vi "ContextManager.FGV.vi"(10 "error in":errorcluster, 11 "action":T1) -> (2 "error out":errorcluster, 3 "context":refnum<class "zmq_context.lvclass">)   [LabVIEW 2019, in "RemoteControl.ZMQ.lvlib" / "ZMQ.ContextManager.lvlib"]
uses:
  ZMQ.ContextManager.lvlib
  <vilib>/addons/zeromq/zmq_context.lvclass
  Typedefs/Action--enum.ctl
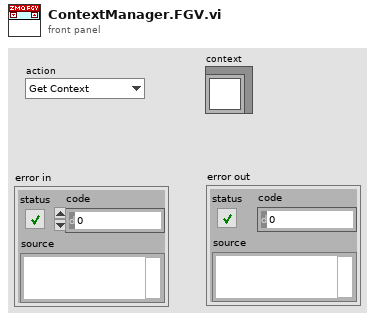
[diagram p1: front panel]
types:
  T1 = typedef "RemoteControl.ZMQ.lvlib/ZMQ.ContextManager.lvlib/Action--enum.ctl" = enum16{"Get Context", "Release Context", "Socket Opened", "Socket Closed", "Force Cleanup"}
  T2 = typedef "RemoteControl.ZMQ.lvlib/ZMQ.ContextManager.lvlib/Context--DVR.ctl" = refnum<data-value>
  T3 = typedef "RemoteControl.ZMQ.lvlib/ZMQ.ContextManager.lvlib/Context--Cluster.ctl" = cluster{"context":refnum<class "zmq_context.lvclass">, "context counter":u32, "socket counter":u32}
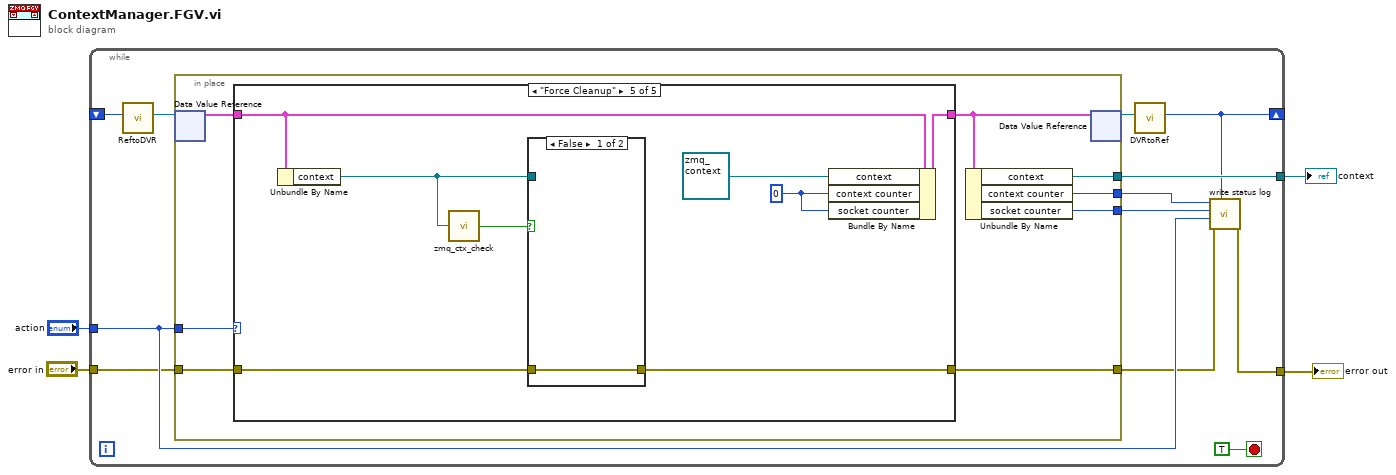
[diagram p0: block diagram]
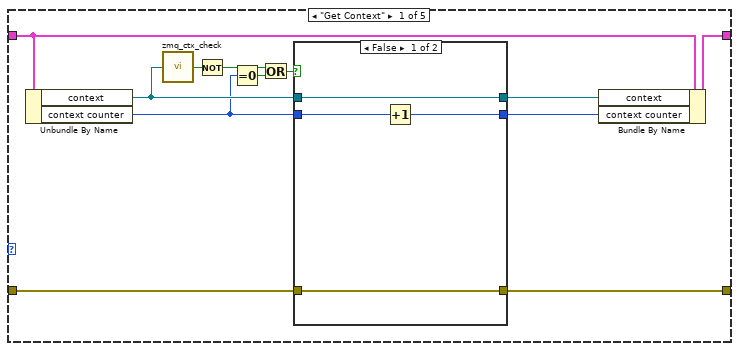
[diagram p2: hidden frame]
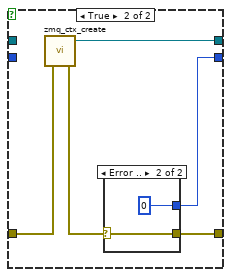
[diagram p3: hidden frame]
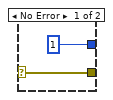
[diagram p4: hidden frame]
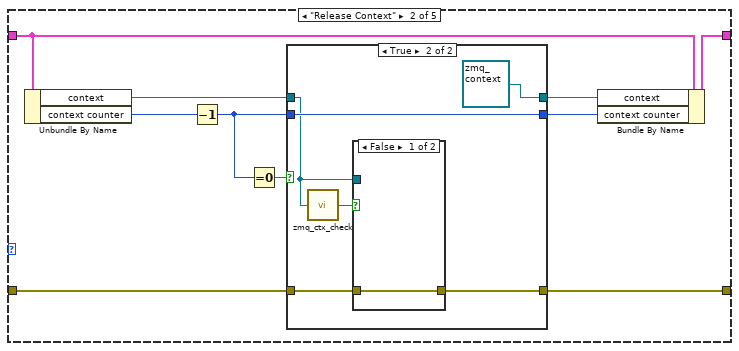
[diagram p5: hidden frame]
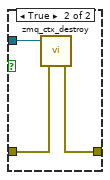
[diagram p7: hidden frame]
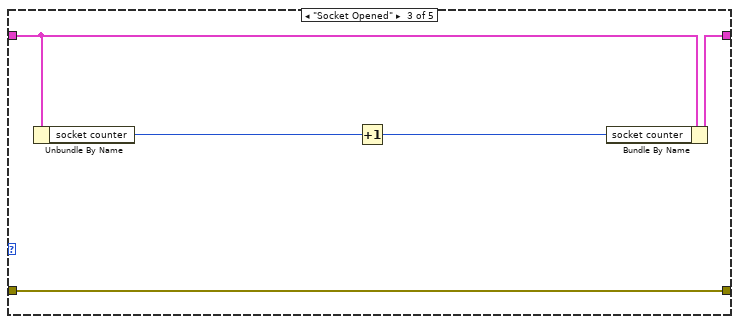
[diagram p8: hidden frame]
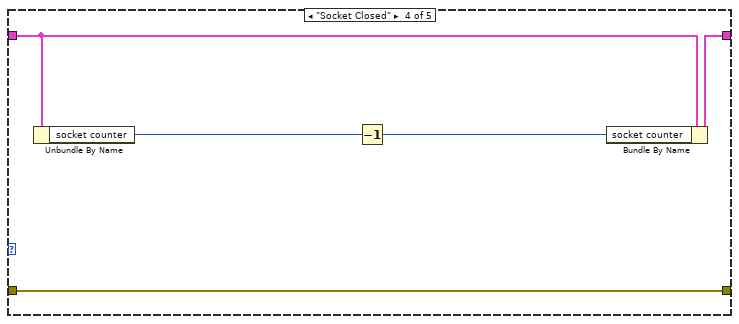
[diagram p9: hidden frame]
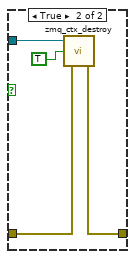
[diagram p10: hidden frame]
diagram:
  n1 = while {
    tunnel: "action" -> [w8]
    shift-right: [w11] -> _
    shift-left: _ -> [w15]
    tunnel: [w12] -> w3
    tunnel: "error in" -> [w7]
    tunnel: [w5] -> w1
    stop <- TRUE stop-if-true
    n2 = call "ReftoDVR.vi"("Ref"=w15) -> ("DVR"=w13:T2)  [unwired: 10 in]
    n3 = in-place {
      in-place-border: [w24] -> w6
      in-place-border: w8 -> [w23]
      in-place-border: [w20] -> w12
      in-place-border: [w19] -> w10
      in-place-border: [w18] -> w9
      in-place-border: w7 -> [w17]
      n4 = in-place-dvr #1(w13) -> (w22:T3)  [unwired: 1 out]
      n5 = case shown="\"Force Cleanup\"" w23 {
        tunnel: w17 -> [w36 w59 w77 w82 w83]
        tunnel: [w35 w58 w77 w82 w90] -> w24
        tunnel: w22 -> [w29 w53 w76 w81 w87]
        tunnel: [w25 w52 w73 w78 w86] -> w21
        frame "Get Context" {
          n6 = Unbundle By Name(w29) -> ("context"=w30:refnum<class "zmq_context.lvclass">, "context counter"=w26:u32)
          n7 = call <vilib>:"zmq_ctx_check.vi"("context in"=w30) -> ("valid?"=w34:bool)
          n8 = Not(x=w34) -> (.not. x?=w31:bool)
          n9 = Equal To 0?(x=w26) -> (x = 0?=w32:bool)
          n10 = Or(x=w31, y=w32) -> (x .or. y?=w33:bool)
          n11 = case shown="False" w33 {
            tunnel: [w37 w45] -> w28
            tunnel: w36 -> [w40 w44]
            tunnel: [w40 w41] -> w35
            tunnel: w26 -> [w39 _]
            tunnel: [w38 w43] -> w27
            tunnel: w30 -> [w37 _]
            frame False {
              n12 = Increment(x=w39) -> (x+1=w38:u32)
            }
            frame True {
              n13 = call <vilib>:"zmq_ctx_create.vi"("error in"=w44) -> ("error out"=w42:errorcluster, "context out"=w45:refnum<class "zmq_context.lvclass">)  [unwired: 3 in]
              n14 = case shown="Error .." w42 {
                selector: w42 -> [w46 w48]
                tunnel: [u32 1 u32 0] -> w43
                tunnel: [w46 w48] -> w41
                frame No Error {
                }
                frame Error {
                }
              }
            }
          }
          n15 = Bundle By Name(cluster=w29, "context"=w28, "context counter"=w27) -> (w25:T3)
        }
        frame "Release Context" {
          n16 = Unbundle By Name(w53) -> ("context"=w50:refnum<class "zmq_context.lvclass">, "context counter"=w51:u32)
          n17 = Decrement(x=w51) -> (x-1=w55:u32)
          n18 = Equal To 0?(x=w55) -> (x = 0?=w57:bool)
          n19 = case shown="True" w57 {
            tunnel: w59 -> [w62 w68]
            tunnel: [w62 w67] -> w58
            tunnel: [w61 refnum<class "zmq_context.lvclass"> refnum ("context out")] -> w54
            tunnel: w50 -> [w61 w63]
            tunnel: [w60 w64] -> w56
            tunnel: w55 -> [w60 w64]
            frame False {
            }
            frame True {
              n20 = call <vilib>:"zmq_ctx_check.vi"("context in"=w63) -> ("valid?"=w66:bool)
              n21 = case shown="False" w66 {
                tunnel: w68 -> [w69 w72]
                tunnel: [w69 w71] -> w67
                tunnel: w63 -> [_ w70]
                frame False {
                }
                frame True {
                  n22 = call <vilib>:"zmq_ctx_destroy.vi"("error in"=w72, "context in"=w70) -> ("error out"=w71:errorcluster)  [unwired: 3 in]
                }
              }
            }
          }
          n23 = Bundle By Name(cluster=w53, "context"=w54, "context counter"=w56) -> (w52:T3)
        }
        frame "Socket Opened" {
          n24 = Unbundle By Name(w76) -> ("socket counter"=w75:u32)
          n25 = Increment(x=w75) -> (x+1=w74:u32)
          n26 = Bundle By Name(cluster=w76, "socket counter"=w74) -> (w73:T3)
        }
        frame "Socket Closed" {
          n27 = Unbundle By Name(w81) -> ("socket counter"=w80:u32)
          n28 = Decrement(x=w80) -> (x-1=w79:u32)
          n29 = Bundle By Name(cluster=w81, "socket counter"=w79) -> (w78:T3)
        }
        frame "Force Cleanup" {
          w85 = u32 0
          n30 = Unbundle By Name(w87) -> ("context"=w84:refnum<class "zmq_context.lvclass">)
          n31 = call <vilib>:"zmq_ctx_check.vi"("context in"=w84) -> ("valid?"=w89:bool)
          n32 = case shown="False" w89 {
            tunnel: w83 -> [w91 w95]
            tunnel: [w91 w94] -> w90
            tunnel: w84 -> [_ w92]
            frame False {
            }
            frame True {
              n33 = call <vilib>:"zmq_ctx_destroy.vi"("error in"=w95, "reap? (F)"=TRUE, "context in"=w92) -> ("error out"=w94:errorcluster)  [unwired: 2 in]
            }
          }
          n34 = Bundle By Name(cluster=w87, "context"=refnum<class "zmq_context.lvclass"> refnum ("context out"), "context counter"=w85, "socket counter"=w85) -> (w86:T3)
        }
      }
      n35 = Unbundle By Name(w21) -> ("context"=w20:refnum<class "zmq_context.lvclass">, "context counter"=w19:u32, "socket counter"=w18:u32)
      n36 = in-place-dvr #1(w21) -> (w14:T2)  [unwired: 1 out]
    }
    n37 = call "DVRtoRef.vi"("DVR"=w14) -> ("Ref"=w11:u32)  [unwired: 10 in]
    n38 = call "write status log.vi"("Context ID"=w11, "error in"=w6, "Action"=w8, "Socket Counter"=w9, "Context Counter"=w10) -> ("error out"=w5:errorcluster)  [unwired: 6 in]
  }
  "context" <- w3
  "error out" <- w1
